vi "Error Converter(ErrCheck).vi"(8 "error in (no error)":errorcluster) -> (0 "error out":errorcluster)   [LabVIEW 2020, in "ASDK.lvlib"]
uses:
  ASDK.lvlib
  ASDK.dll
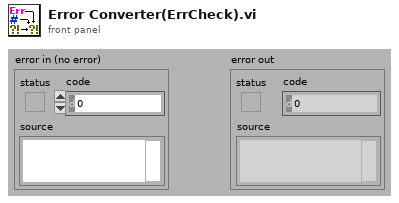
[diagram p1: front panel]
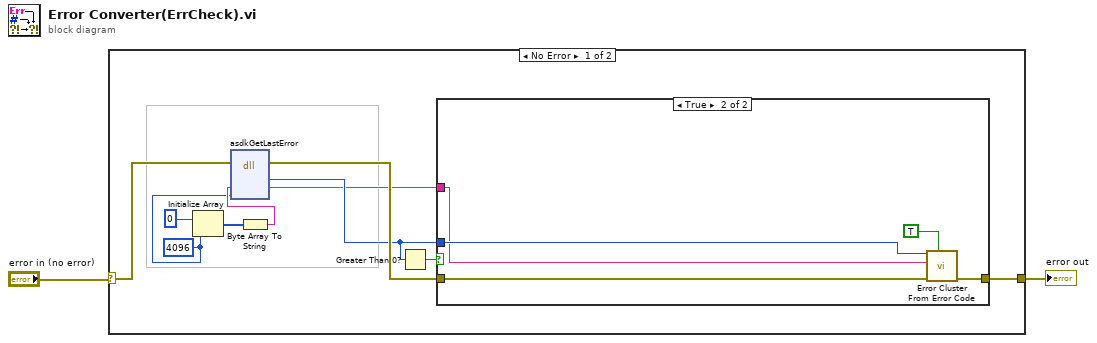
[diagram p0: block diagram]
diagram:
  n1 = case shown="No Error" "error in (no error)" {
    selector: "error in (no error)" -> [w10 w19]
    tunnel: [w11 w19] -> w1
    frame No Error {
      w3 = 4096 ("dimension size")
      n2 = Initialize Array(u8 0 ("element"), w3) -> (w6:u8[])
      n3 = Byte Array To String(unsigned byte array=w6) -> (string=w4:string)
      n4 = dll-call lib="ASDK.*" fn="asdkGetLastError"(error in=w10, "errMsg"=w4, "errSize"=w3) -> (error out=w9:errorcluster, "errorNo"=w8:u32, "errMsg"=w7:string)  [unwired: 5 in, 1 out]
      n5 = Greater Than 0?(x=w8) -> (x > 0?=w12:bool)
      n6 = case shown="True" w12 {
        tunnel: w9 -> [w13 w16]
        tunnel: w8 -> [_ w17]
        tunnel: [w13 w15] -> w11
        tunnel: w7 -> [_ w14]
        frame False {
        }
        frame True {
          n7 = call <vilib>:"Error Cluster From Error Code.vi"("show call chain? (False)"=TRUE, "error in (no error)"=w16, "error message (\"\")"=w14, "error code (0)"=w17) -> ("error out"=w15:errorcluster)  [unwired: 5 in]
        }
      }
    }
    frame Error {
    }
  }
  "error out" <- w1
